vi "Write plots names.vi"(8 "error in (no error)":errorcluster, 9 "Combo Box":string(combo)="Kinetics", 10 "Plot names":string[](array[string])=["part", "full"], 11 "Control-Client in":refnum<class "Control-Client.lvclass">) -> (0 "error out":errorcluster, 3 "Control-Client out":refnum<class "Control-Client.lvclass">)   [LabVIEW 2018, in "Control-Client.lvclass"]
uses:
  Control-Client.lvclass
  Control-Client.lvclass/Control-Client.ctl
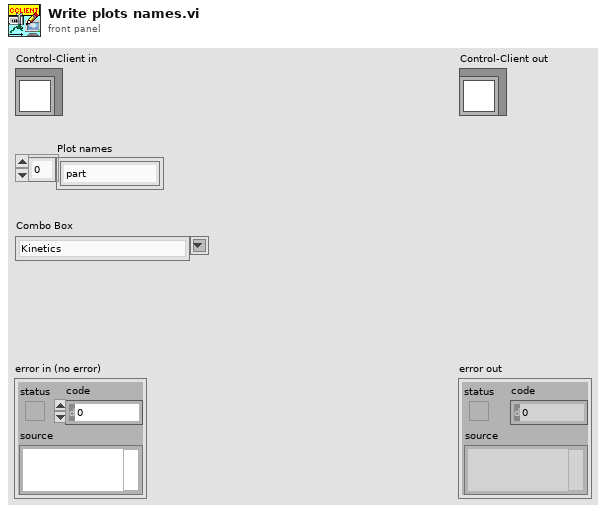
[diagram p1: front panel]
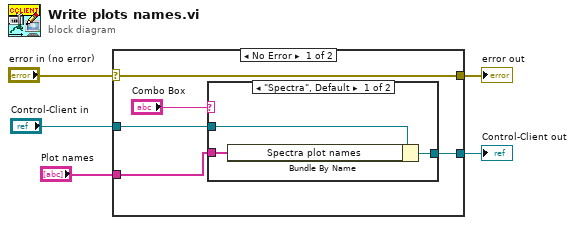
[diagram p0: block diagram]
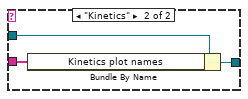
[diagram p2: hidden frame]
diagram:
  n1 = case shown="No Error" "error in (no error)" {
    selector: "error in (no error)" -> [w10 w17]
    tunnel: [w10 w17] -> w4
    tunnel: [w8 w18] -> w2
    tunnel: "Control-Client in" -> [w9 w18]
    tunnel: "Plot names" -> [w7 _]
    frame No Error {
      n2 = case shown="\"Spectra\", Default" "Combo Box" {
        tunnel: w9 -> [w12 w16]
        tunnel: [w11 w15] -> w8
        tunnel: w7 -> [w13 w14]
        frame "Spectra", Default {
          n3 = Bundle By Name(cluster=w12, "Spectra plot names"=w13) -> (w11:refnum<class "Control-Client.lvclass">)
        }
        frame "Kinetics" {
          n4 = Bundle By Name(cluster=w16, "Kinetics plot names"=w14) -> (w15:refnum<class "Control-Client.lvclass">)
        }
      }
    }
    frame Error {
    }
  }
  "error out" <- w4
  "Control-Client out" <- w2
